vi "Coincident points test.vi"(1 "epsilon":sgl, 2 "Point 2":sgl[](array[numeric]), 3 "Point 1":sgl[](array[numeric])) -> (0 "Points are coincident":bool)   [LabVIEW 2014]
panel:
  # "PN 21/03/2015"
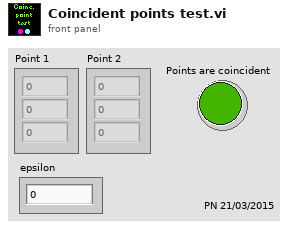
[diagram p1: front panel]
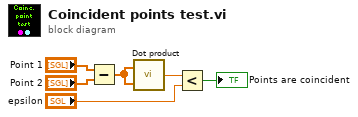
[diagram p0: block diagram]
diagram:
  n1 = Subtract(x="Point 1", y="Point 2") -> (x-y=w1:sgl[])
  n2 = call "Dot product.vi"("B"=w1, "A"=w1) -> ("A . B"=w6:sgl)
  n3 = Less?(x=w6, y="epsilon") -> (x < y?=→"Points are coincident":bool)
